vi "Build Image Array (SubVI).vi"(10 "Image Pixels (U8) in":u8[][](array[numeric]), 11 "Rows (X)":u16) -> (2 "Image Pixels B (U8) 3":u8[](array[numeric]), 3 "Image Pixels A (U8) out":u8[](array[numeric]))   [LabVIEW 2017]
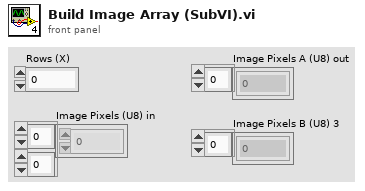
[diagram p1: front panel]
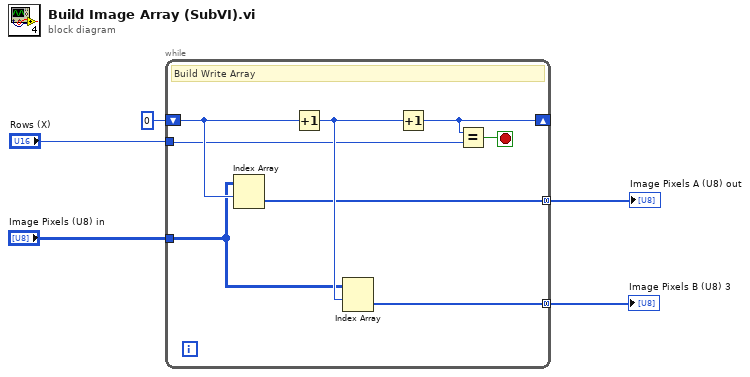
[diagram p0: block diagram]
diagram:
  n1 = while {
    shift-right: [w11] -> _
    shift-left: 0 ("y") -> [w13]
    tunnel: "Rows (X)" -> [w9]
    tunnel: [w8] -> w2 mode=concatenating
    tunnel: [w7] -> w3 mode=concatenating
    tunnel: "Image Pixels (U8) in" -> [w6]
    stop <- w10 stop-if-true
    # "Build Write Array"
    n2 = Index Array(array=w6, index (row)=w13) -> (element=w7:u8[])  [unwired: 1 in]
    n3 = Increment(x=w13) -> (x+1=w12:i32)
    n4 = Index Array(array=w6, index (row)=w12) -> (element=w8:u8[])  [unwired: 1 in]
    n5 = Increment(x=w12) -> (x+1=w11:i32)
    n6 = Equal?(x=w11, y=w9) -> (x = y?=w10:bool)
  }
  "Image Pixels A (U8) out" <- w3
  "Image Pixels B (U8) 3" <- w2
